vi "PushTiles.vi"(8 "error in (no error)":errorcluster, 10 "Refnum in":T5, 11 "TilesLoopData in":T1) -> (0 "error out":errorcluster, 3 "TilesLoopData out":T1)   [LabVIEW 2019, in "RT_Game.lvlib" / "Engine.lvclass"]
uses:
  Engine.lvclass
  TilesLoopData.ctl
  Game/Coordinate.ctl
  Game/SlideJob.ctl
  Game/ScreenSide.ctl
  FPGA_Interface.ctl
  <vilib>/Utility/error.llb/Error Cluster From Error Code.vi
  <vilib>/rvi/errors/niLvFpgaAdjustHostInterfaceError.vi
  <vilib>/rvi/interface/nirviMethod/nirviMethod.xnode
  FPGA Bitfiles/myriogameconsole_FPGATarget_Main_ntsPRcBZGxk.lvbitx
  <vilib>/FPGAPlugInAG/myRIO-1900/niLvFpga_WriteFifo_myRIO-1900.vi
  <vilib>/rvi/errors/niLvFpgaMergeErrorWithErrorCode.vi
  Game/Game.lvclass
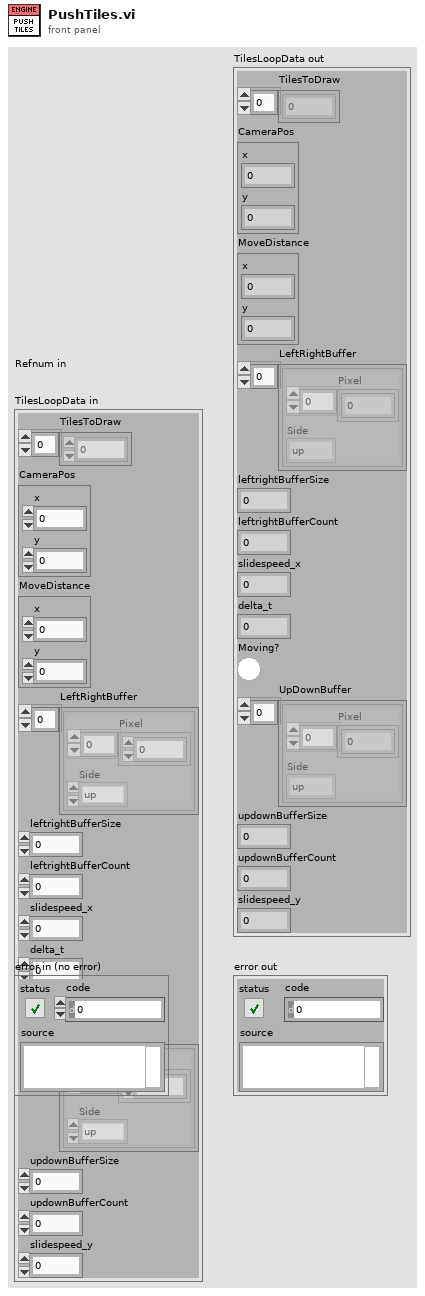
[diagram p1: front panel]
types:
  T1 = typedef "RT_Game.lvlib/Engine.lvclass/TilesLoopData.ctl" = cluster{"TilesToDraw":u64[], "CameraPos":T2, "MoveDistance":T2, "LeftRightBuffer":T3[], "leftrightBufferSize":i16, "leftrightBufferCount":i16, "slidespeed_x":dbl, "delta_t":dbl, "Moving?":bool, "UpDownBuffer":T3[], "updownBufferSize":i16, "updownBufferCount":i16, "slidespeed_y":dbl}
  T2 = typedef "RT_Game.lvlib/Game.lvclass/Coordinate.ctl" = cluster{"x":dbl, "y":dbl}
  T3 = typedef "RT_Game.lvlib/Engine.lvclass/SlideJob.ctl" = cluster{"Pixel":u32[], "Side":T4}
  T4 = typedef "RT_Game.lvlib/Game.lvclass/ScreenSide.ctl" = enum16{"up", "down", "left", "right", "none"}
  T5 = typedef "FPGA_Interface.ctl" = refnum<k20>
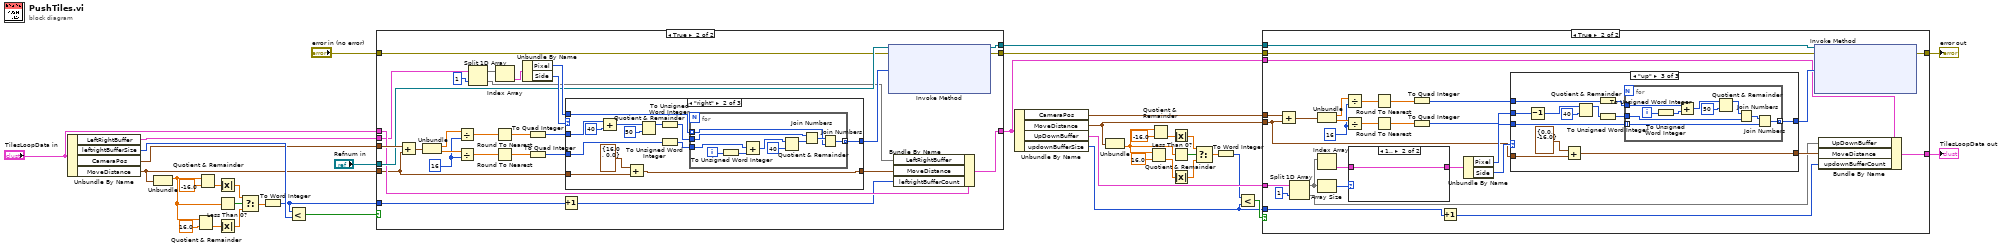
[diagram p0: block diagram]
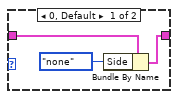
[diagram p3: hidden frame]
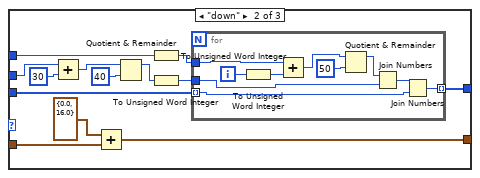
[diagram p5: hidden frame]
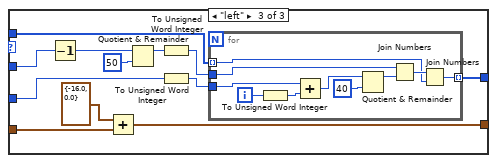
[diagram p8: hidden frame]
diagram:
  n1 = Unbundle By Name("TilesLoopData in") -> ("LeftRightBuffer"=w38:T3[], "leftrightBufferSize"=w37:i16, "CameraPos"=w12:T2, "MoveDistance"=w11:T2)
  n2 = Unbundle(w11) -> ("x"=w25:dbl)  [unwired: 1 out]
  n3 = Quotient & Remainder(x=w25, y=16.0) -> (floor(x/y)=w32:dbl)  [unwired: 1 out]
  n4 = Quotient & Remainder(x=w25, y=-16.0) -> (floor(x/y)=w27:dbl)  [unwired: 1 out]
  n5 = Absolute Value(x=w27) -> (abs(x)=w24:dbl)
  n6 = Less Than 0?(x=w25) -> (x < 0?=w28:bool)
  n7 = Absolute Value(x=w32) -> (abs(x)=w30:dbl)
  n8 = Select(t=w24, s=w28, f=w30) -> (s? t:f=w29:dbl)
  n9 = To Word Integer(number=w29) -> (16bit integer=w31:i16)
  n10 = Less?(x=w31, y=w37) -> (x < y?=w34:bool)
  n11 = case shown="True" w34 {
    tunnel: w12 -> [_ w69]
    tunnel: w38 -> [_ w52]
    tunnel: [w40 w68] -> w6
    tunnel: "Refnum in" -> [w39 w60]
    tunnel: [w41 w59] -> w13
    tunnel: "TilesLoopData in" -> [w40 w58]
    tunnel: "error in (no error)" -> [w41 w57]
    tunnel: w31 -> [_ w55]
    tunnel: w11 -> [_ w43]
    tunnel: [w39 w42] -> w7
    frame False {
    }
    frame True {
      w47 = u16 16 ("y")
      n12 = Add(x=w69, y=w43) -> (x+y=w53:T2)
      n13 = Unbundle(w53) -> ("x"=w46:dbl, "y"=w64:dbl)
      n14 = Divide(x=w46, y=w47) -> (x/y=w45:dbl)
      n15 = Divide(x=w64, y=w47) -> (x/y=w48:dbl)
      n16 = Split 1D Array(array=w52, index=1) -> (first subarray=w49:T3[], second subarray=w50:T3[])
      n17 = Round To Nearest(number=w45) -> (nearest integer value=w44:dbl)
      n18 = Round To Nearest(number=w48) -> (nearest integer value=w63:dbl)
      n19 = Index Array(array=w49) -> (element=w67:T3)  [unwired: 1 in]
      n20 = Unbundle By Name(w67) -> ("Pixel"=w65:u32[], "Side"=w66:T4)
      n21 = To Quad Integer(1:w44) -> (0:w61:i64)
      n22 = To Quad Integer(1:w63) -> (0:w62:i64)
      n23 = Increment(x=w55) -> (x+1=w54:i16)
      n24 = case shown="\"right\"" w66 {
        tunnel: w61 -> [_ w77 w101]
        tunnel: w62 -> [_ w76 w100]
        tunnel: w65 -> [_ w75 w99]
        tunnel: w43 -> [w71 w74 w98]
        tunnel: [w71 w73 w97] -> w56
        tunnel: [_ w72 w96] -> w70
        frame Default {
        }
        frame "right" {
          n25 = Add(x=w77, y=u16 40) -> (x+y=w83:i64)
          n26 = Add(x=T2 {"x"=16.0, "y"=0.0}, y=w74) -> (x+y=w73:T2)
          n27 = Quotient & Remainder(x=w83, y=u16 50) -> (x-y*floor(x/y)=w81:i64)  [unwired: 1 out]
          n28 = To Unsigned Word Integer(number=w81) -> (unsigned 16bit integer=w80:u16)
          n29 = To Unsigned Word Integer(number=w76) -> (unsigned 16bit integer=w79:u16)
          n30 = for {
            tunnel: w79 -> [w92]
            tunnel: w80 -> [w86]
            tunnel: [w88] -> w72 mode=indexing
            tunnel: w75 -> [w87] mode=indexing
            i -> [w93]
            n31 = To Unsigned Word Integer(number=w93) -> (unsigned 16bit integer=w89:u16)
            n32 = Add(x=w92, y=w89) -> (x+y=w90:u16)
            n33 = Quotient & Remainder(x=w90, y=u16 40) -> (x-y*floor(x/y)=w85:u16)  [unwired: 1 out]
            n34 = Join Numbers(hi=w86, lo=w85) -> ((hi.lo)=w94:u32)
            n35 = Join Numbers(hi=w94, lo=w87) -> ((hi.lo)=w88:u64)
          }
        }
        frame "left" {
          n36 = Decrement(x=w101) -> (x-1=w95:i64)
          n37 = Add(x=T2 {"x"=-16.0, "y"=0.0}, y=w98) -> (x+y=w97:T2)
          n38 = Quotient & Remainder(x=w95, y=u16 50) -> (x-y*floor(x/y)=w105:i64)  [unwired: 1 out]
          n39 = To Unsigned Word Integer(number=w105) -> (unsigned 16bit integer=w104:u16)
          n40 = To Unsigned Word Integer(number=w100) -> (unsigned 16bit integer=w103:u16)
          n41 = for {
            tunnel: w103 -> [w114]
            tunnel: w104 -> [w113]
            tunnel: [w108] -> w96 mode=indexing
            tunnel: w99 -> [w107] mode=indexing
            i -> [w115]
            n42 = To Unsigned Word Integer(number=w115) -> (unsigned 16bit integer=w109:u16)
            n43 = Add(x=w114, y=w109) -> (x+y=w111:u16)
            n44 = Quotient & Remainder(x=w111, y=u16 40) -> (x-y*floor(x/y)=w110:u16)  [unwired: 1 out]
            n45 = Join Numbers(hi=w113, lo=w110) -> ((hi.lo)=w116:u32)
            n46 = Join Numbers(hi=w116, lo=w107) -> ((hi.lo)=w108:u64)
          }
        }
      }
      n47 = xnode "Invoke Method"("FPGA VI Reference In"=w60, "error in"=w57, "Data"=w70) -> ("FPGA VI Reference Out"=w42:T5, "error out"=w59:errorcluster)  [unwired: 1 in, 1 out]
      n48 = Bundle By Name(cluster=w58, "LeftRightBuffer"=w50, "MoveDistance"=w56, "leftrightBufferCount"=w54) -> (w68:T1)
    }
  }
  n49 = Unbundle By Name(w6) -> ("CameraPos"=w5:T2, "MoveDistance"=w2:T2, "UpDownBuffer"=w4:T3[], "updownBufferSize"=w1:i16)
  n50 = Unbundle(w2) -> ("y"=w8:dbl)  [unwired: 1 out]
  n51 = Quotient & Remainder(x=w8, y=16.0) -> (floor(x/y)=w17:dbl)  [unwired: 1 out]
  n52 = Quotient & Remainder(x=w8, y=-16.0) -> (floor(x/y)=w21:dbl)  [unwired: 1 out]
  n53 = Absolute Value(x=w21) -> (abs(x)=w23:dbl)
  n54 = Less Than 0?(x=w8) -> (x < 0?=w20:bool)
  n55 = Absolute Value(x=w17) -> (abs(x)=w18:dbl)
  n56 = Select(t=w23, s=w20, f=w18) -> (s? t:f=w19:dbl)
  n57 = To Word Integer(number=w19) -> (16bit integer=w3:i16)
  n58 = Less?(x=w3, y=w1) -> (x < y?=w15:bool)
  n59 = case shown="True" w15 {
    tunnel: w5 -> [_ w147]
    tunnel: w4 -> [_ w130]
    tunnel: [w117 w146] -> w9
    tunnel: w7 -> [_ w138]
    tunnel: [w118 w137] -> w10
    tunnel: w6 -> [w117 w136]
    tunnel: w13 -> [w118 w135]
    tunnel: w1 -> [_ w133]
    tunnel: w2 -> [_ w122]
    frame False {
    }
    frame True {
      w126 = u16 16 ("y")
      n60 = Add(x=w147, y=w122) -> (x+y=w131:T2)
      n61 = Split 1D Array(array=w130, index=1) -> (first subarray=w120:T3[], second subarray=w128:T3[])
      n62 = Unbundle(w131) -> ("x"=w125:dbl, "y"=w142:dbl)
      n63 = Index Array(array=w120) -> (element=w145:T3)  [unwired: 1 in]
      n64 = Array Size(array=w120) -> (size(s)=w119:i32)
      n65 = Divide(x=w125, y=w126) -> (x/y=w124:dbl)
      n66 = Divide(x=w142, y=w126) -> (x/y=w127:dbl)
      n67 = case shown="1.." w119 {
        tunnel: w145 -> [w151 w152]
        tunnel: [w150 w152] -> w121
        frame 0, Default {
          n68 = Bundle By Name(cluster=w151, "Side"=ScreenSide."none") -> (w150:T3)
        }
        frame 1.. {
        }
      }
      n69 = Round To Nearest(number=w124) -> (nearest integer value=w123:dbl)
      n70 = Round To Nearest(number=w127) -> (nearest integer value=w141:dbl)
      n71 = To Quad Integer(1:w123) -> (0:w139:i64)
      n72 = To Quad Integer(1:w141) -> (0:w140:i64)
      n73 = Increment(x=w133) -> (x+1=w132:i16)
      n74 = Unbundle By Name(w121) -> ("Pixel"=w143:u32[], "Side"=w144:T4)
      n75 = case shown="\"up\"" w144 {
        tunnel: w139 -> [_ w154 w177]
        tunnel: w140 -> [_ w156 w179]
        tunnel: w143 -> [_ w160 w184]
        tunnel: w122 -> [w153 w159 w183]
        tunnel: [w153 w158 w182] -> w134
        tunnel: [_ w157 w181] -> w148
        frame Default {
        }
        frame "down" {
          n76 = Add(x=w156, y=u16 30) -> (x+y=w165:i64)
          n77 = Add(x=T2 {"x"=0.0, "y"=16.0}, y=w159) -> (x+y=w158:T2)
          n78 = Quotient & Remainder(x=w165, y=u16 40) -> (x-y*floor(x/y)=w155:i64)  [unwired: 1 out]
          n79 = To Unsigned Word Integer(number=w154) -> (unsigned 16bit integer=w163:u16)
          n80 = To Unsigned Word Integer(number=w155) -> (unsigned 16bit integer=w162:u16)
          n81 = for {
            tunnel: w162 -> [w167]
            tunnel: w163 -> [w169]
            tunnel: [w171] -> w157 mode=indexing
            tunnel: w160 -> [w170] mode=indexing
            i -> [w175]
            n82 = To Unsigned Word Integer(number=w175) -> (unsigned 16bit integer=w172:u16)
            n83 = Add(x=w169, y=w172) -> (x+y=w173:u16)
            n84 = Quotient & Remainder(x=w173, y=u16 50) -> (x-y*floor(x/y)=w168:u16)  [unwired: 1 out]
            n85 = Join Numbers(hi=w168, lo=w167) -> ((hi.lo)=w176:u32)
            n86 = Join Numbers(hi=w176, lo=w170) -> ((hi.lo)=w171:u64)
          }
        }
        frame "up" {
          n87 = Decrement(x=w179) -> (x-1=w180:i64)
          n88 = Add(x=T2 {"x"=0.0, "y"=-16.0}, y=w183) -> (x+y=w182:T2)
          n89 = Quotient & Remainder(x=w180, y=u16 40) -> (x-y*floor(x/y)=w178:i64)  [unwired: 1 out]
          n90 = To Unsigned Word Integer(number=w177) -> (unsigned 16bit integer=w187:u16)
          n91 = To Unsigned Word Integer(number=w178) -> (unsigned 16bit integer=w186:u16)
          n92 = for {
            tunnel: w186 -> [w189]
            tunnel: w187 -> [w191]
            tunnel: [w193] -> w181 mode=indexing
            tunnel: w184 -> [w192] mode=indexing
            i -> [w197]
            n93 = To Unsigned Word Integer(number=w197) -> (unsigned 16bit integer=w194:u16)
            n94 = Add(x=w191, y=w194) -> (x+y=w195:u16)
            n95 = Quotient & Remainder(x=w195, y=u16 50) -> (x-y*floor(x/y)=w190:u16)  [unwired: 1 out]
            n96 = Join Numbers(hi=w190, lo=w189) -> ((hi.lo)=w198:u32)
            n97 = Join Numbers(hi=w198, lo=w192) -> ((hi.lo)=w193:u64)
          }
        }
      }
      n98 = xnode "Invoke Method"("FPGA VI Reference In"=w138, "error in"=w135, "Data"=w148) -> ("error out"=w137:errorcluster)  [unwired: 1 in, 2 out]
      n99 = Bundle By Name(cluster=w136, "UpDownBuffer"=w128, "MoveDistance"=w134, "updownBufferCount"=w132) -> (w146:T1)
    }
  }
  "TilesLoopData out" <- w9
  "error out" <- w10
